vi "Extract XML data LV 8_6.vi"() -> ()   [LabVIEW 2011]
panel:
  out "value":cluster{string, string}
  out "text":string
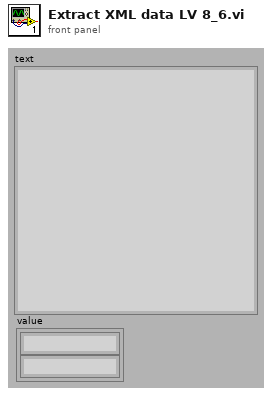
[diagram p1: front panel]
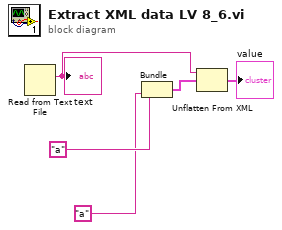
[diagram p0: block diagram]
diagram:
  n1 = Read from Text File() -> (text=w5:string)  [unwired: 4 in, 3 out]
  "text" <- w5
  n2 = Bundle("a", "a") -> (w3:cluster{string, string})  [unwired: 1 in]
  n3 = Unflatten From XML(xml string=w5, type=w3) -> (value=→"value":cluster{string, string})  [unwired: 1 in, 1 out]
